vi "Write Value (variant).vi"(8 "error in (no error)":errorcluster, 10 "Variant":variant, 11 "String D Element in":refnum<class "String D Element.lvclass">) -> (0 "error out":errorcluster, 3 "String D Element out":refnum<class "String D Element.lvclass">)   [LabVIEW 2018, in "D Datagrid Library.lvlib" / "String D Element.lvclass"]
uses:
  String D Element.lvclass
  String D Element.lvclass/String D Element.ctl
  Write Value.vi
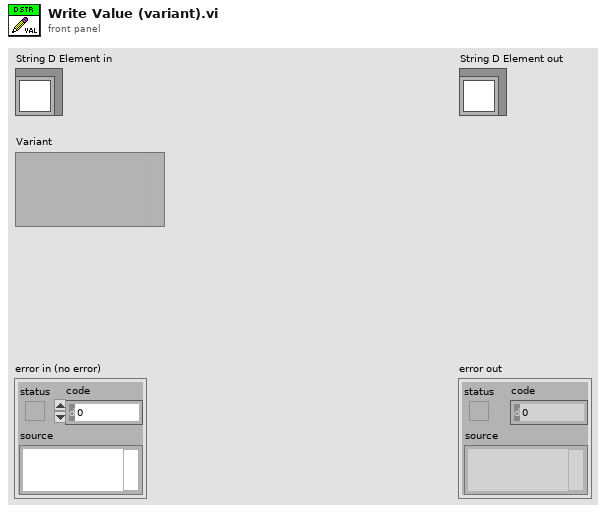
[diagram p1: front panel]
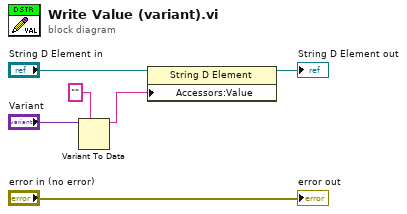
[diagram p0: block diagram]
diagram:
  n1 = Variant To Data(type="" ("Value"), Variant="Variant") -> (data=w3:string)  [unwired: 1 in, 1 out]
  n2 = property class="String D Element"(reference="String D Element in", "Accessors:Value"=w3) -> (reference out=→"String D Element out":refnum<class "String D Element.lvclass">)  [unwired: 1 in, 1 out]
  "error out" <- "error in (no error)"
